vi "SS2 Live_Upload Bitfile.vi"(8 "error in (no error)":errorcluster, 10 "FPGA bitfile Path":path, 11 "okCFrontPanel Device Refnum":refnum<k24>) -> (0 "error out":errorcluster, 3 "okCFrontPanel Device Refnum":refnum<k24>)   [LabVIEW 2019]
uses:
  C:/UCLA Thinkpad Google Drive/LabVIEW 2019 SP1/builds/SS2 Live Distribution/Opal Kelly/C# Wrapper/libFrontPanel-csharp.dll
  Opal Kelly/C# Wrapper/libFrontPanel-csharp.dll
  Opal Kelly/C# Wrapper/okFrontPanelC#Wrapper.lvlib
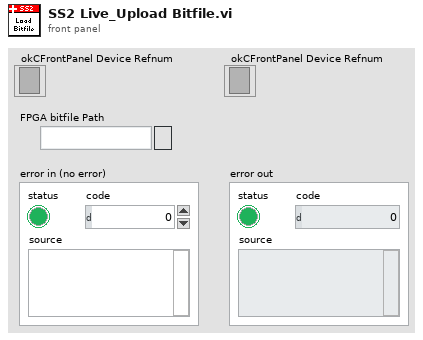
[diagram p1: front panel]
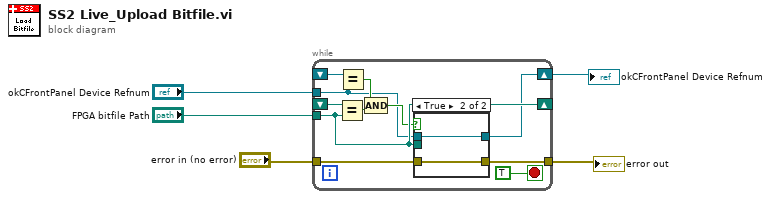
[diagram p0: block diagram]
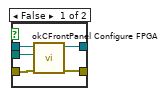
[diagram p2: hidden frame]
diagram:
  n1 = while {
    tunnel: "FPGA bitfile Path" -> [w13]
    tunnel: "okCFrontPanel Device Refnum" -> [w6]
    shift-right: [w7] -> w1
    shift-left: _ -> [w15]
    shift-right: [w13] -> _
    shift-left: _ -> [w14]
    tunnel: "error in (no error)" -> [w12]
    tunnel: [w11] -> w2
    stop <- TRUE stop-if-true
    n2 = Equal?(x=w14, y=w13) -> (x = y?=w10:bool)
    n3 = Equal?(x=w15, y=w6) -> (x = y?=w9:bool)
    n4 = Compound Arithmetic op=AND(w9, w10) -> (w8:bool)
    n5 = case shown="True" w8 {
      tunnel: w13 -> [w21 _]
      tunnel: w12 -> [w20 w23]
      tunnel: [w19 w23] -> w11
      tunnel: w6 -> [w18 w22]
      tunnel: [w17 w22] -> w7
      frame False {
        n6 = call "okCFrontPanel Configure FPGA.vi"("error in (no error)"=w20, "FPGA bitfile Path"=w21, "okCFrontPanel Device Refnum"=w18) -> ("error out"=w19:errorcluster, "okCFrontPanel Device Refnum"=w17:refnum<k24>)  [unwired: 7 in]
      }
      frame True {
      }
    }
  }
  "okCFrontPanel Device Refnum" <- w1
  "error out" <- w2
